vi "TCP Engine Hardware Info JSON Conversion.vi"(8 "error in":errorcluster, 11 "JSON String":string) -> (0 "error out":errorcluster, 2 "Sub Command":string, 3 "Command":string)   [LabVIEW 2018, in "TCP Engine.lvlib"]
doc: "All Rights Reserved © 2017 SyncSols"
uses:
  TCP Engine.lvlib
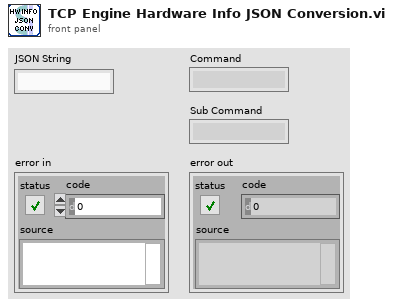
[diagram p1: front panel]
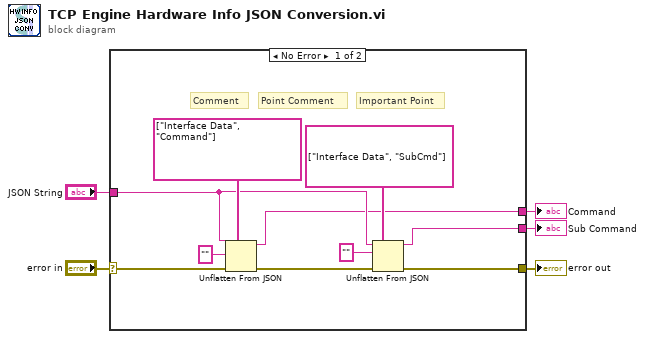
[diagram p0: block diagram]
diagram:
  n1 = case shown="No Error" "error in" {
    selector: "error in" -> [w9 w16]
    tunnel: [w8 w16] -> w5
    tunnel: "JSON String" -> [w10 _]
    tunnel: [w7 _] -> w2
    tunnel: [w6 _] -> w1
    frame No Error {
      # "Important Point"
      # "Point Comment"
      # "Comment"
      n2 = Unflatten From JSON(path=string[] ["Interface Data", "Command"], JSON string=w10, type and defaults="", error in (no error)=w9) -> (value=w7:string, error out=w13:errorcluster)  [unwired: 3 in]
      n3 = Unflatten From JSON(path=string[] ["Interface Data", "SubCmd"], JSON string=w10, type and defaults="", error in (no error)=w13) -> (value=w6:string, error out=w8:errorcluster)  [unwired: 3 in]
    }
    frame Error {
    }
  }
  "error out" <- w5
  "Command" <- w2
  "Sub Command" <- w1
